vi "Create Album.vi"(7 "Songs":refnum<class "Song.lvclass">[](array[class]), 8 "error in (no error)":errorcluster, 9 "Artist Name":string, 10 "Album Name":string, 11 "Album In":refnum<class "Album.lvclass">) -> (0 "error out":errorcluster, 3 "Album out":refnum<class "Album.lvclass">)   [LabVIEW 2015, in "Album.lvclass"]
uses:
  Album.lvclass
  Song/Song.lvclass
  Album.lvclass/Album.ctl
  Write Artist.vi
  Write SongLibrary.vi
  MusicElementLibrary/SongLibrary/SongLibrary.lvclass
  MusicElement.lvclass
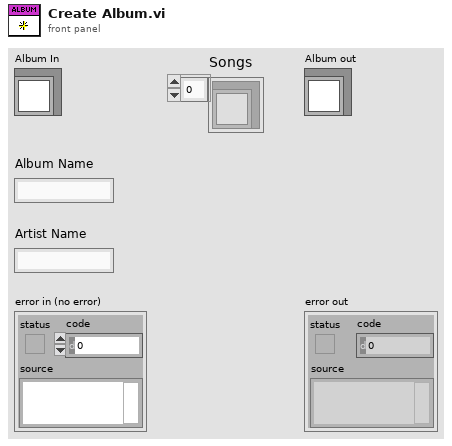
[diagram p1: front panel]
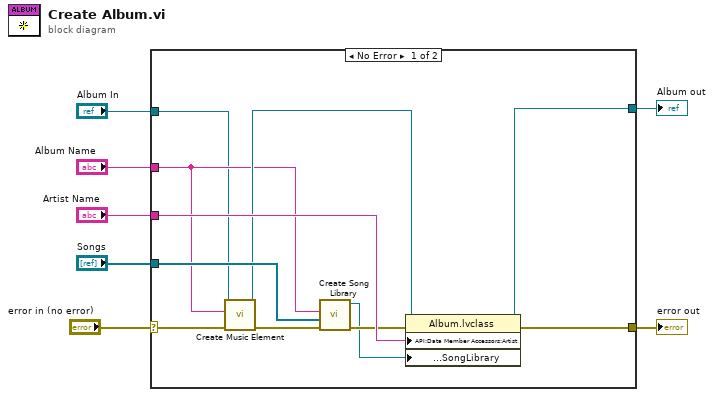
[diagram p0: block diagram]
diagram:
  n1 = case shown="No Error" "error in (no error)" {
    selector: "error in (no error)" -> [w12 w19]
    tunnel: [w18 w19] -> w6
    tunnel: "Artist Name" -> [w16 _]
    tunnel: [w17 _] -> w4
    tunnel: "Album Name" -> [w9 _]
    tunnel: "Songs" -> [w15 _]
    tunnel: "Album In" -> [w8 _]
    frame No Error {
      n2 = call "Create Music Element.vi"("error in (no error)"=w12, "Name"=w9, "MusicElement in"=w8) -> ("error out"=w10:errorcluster, "MusicElement out"=w11:refnum<class "Album.lvclass">)  [unwired: 7 in]
      n3 = call "Create Song Library.vi"("error in (no error)"=w10, "Songs"=w15, "Name"=w9) -> ("error out"=w14:errorcluster, "SongLibrary out"=w13:refnum<class "SongLibrary.lvclass">)  [unwired: 7 in]
      n4 = property class="Album.lvclass"(reference=w11, error in=w14, "API:Data Member Accessors:Artist"=w16, "API:Data Member Accessors:SongLibrary"=w13) -> (reference out=w17:refnum<class "Album.lvclass">, error out=w18:errorcluster)
    }
    frame Error {
    }
  }
  "error out" <- w6
  "Album out" <- w4
